vi "SetHFLockIn.vi"(0 "HF Lockin Cluster":T1={"Amplitude"=-inf, "Phase Shift"=-inf, "Frequency"=-inf, "Integration Time"=-inf, "Sensitivity"=-inf} {"Sensitivity" format="%#_g V"; "Integration Time" format="%#_g µs"; "Frequency" format="%#_g kHz"; "Phase Shift" format="%#_g deg"; "Amplitude" format="%#_g V"}, 5 "error in":T2) -> (14 "Output Cluster":T1={"Amplitude"=-inf, "Phase Shift"=-inf, "Frequency"=-inf, "Integration Time"=-inf, "Sensitivity"=-inf} {"Sensitivity" format="%#_g V"; "Integration Time" format="%#_g µs"; "Frequency" format="%#_g kHz"; "Phase Shift" format="%#_g deg"; "Amplitude" format="%#_g V"}, 19 "error out":T2)   [LabVIEW 2016]
doc: "Sets all parameters relevant to the high frequency lock in. The input cluster contains:\n- Amplitude in V (float) [0 to 10]\n- Frequency in kHz (float) [0 to 2000]\n- Sensitivity in V (float) [0 to 20]\n- Phase Shift in deg (float) [0 to 360]\n- Integration Time in us (float) [1 to 1000000]\nBy passing -Inf (float) or -2147483648 (integer) as input values, the corresponding parameter(s) will be read out."
uses:
  Controls/HF-Lockin_Parameters.ctl
  Controls/Error_Out.ctl
  Files_ASC500/DLL/ASC500_RemoteControlV27.dll
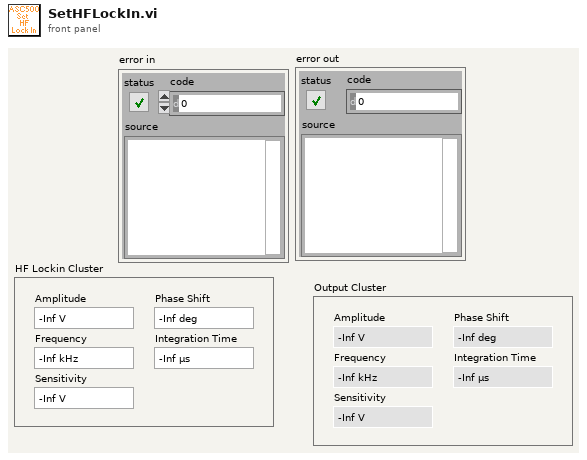
[diagram p1: front panel]
types:
  T1 = typedef "HF-Lockin_Parameters.ctl" = cluster{"Amplitude":sgl, "Phase Shift":sgl, "Frequency":sgl, "Integration Time":sgl, "Sensitivity":sgl}
  T2 = typedef "Error_Out.ctl" = errorcluster
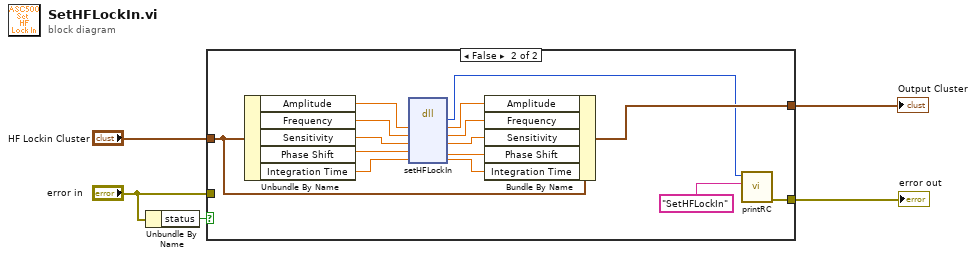
[diagram p0: block diagram]
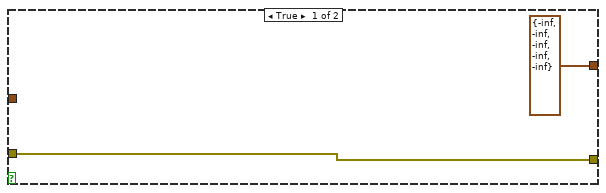
[diagram p2: hidden frame]
diagram:
  n1 = Unbundle By Name("error in") -> ("status"=w5:bool)
  n2 = case shown="False" w5 {
    tunnel: [w6 w10] -> w4
    tunnel: "HF Lockin Cluster" -> [_ w12]
    tunnel: [T1 {"Amplitude"=-inf, "Phase Shift"=-inf, "Frequency"=-inf, "Integration Time"=-inf, "Sensitivity"=-inf} ("HF Lockin Cluster") w11] -> w2
    tunnel: "error in" -> [w6 _]
    frame True {
    }
    frame False {
      n3 = Unbundle By Name(w12) -> ("Amplitude"=w18:sgl, "Frequency"=w19:sgl, "Sensitivity"=w20:sgl, "Phase Shift"=w21:sgl, "Integration Time"=w22:sgl)
      n4 = dll-call lib="G:/SCMOperations/Share/ELE/Produkt Information/ASC500/04 Remote Control/02 development versions/2018Nov06/Files_ASC500/DLL/ASC500_RemoteControlV27.dll" fn="setHFLockIn"("Amplitude"=w18, "Frequency"=w19, "Sensitivity"=w20, "Phase Shift"=w21, "Integration Time"=w22) -> ("return type"=w9:i32, "Amplitude"=w17:sgl, "Frequency"=w16:sgl, "Sensitivity"=w15:sgl, "Phase Shift"=w14:sgl, "Integration Time"=w13:sgl)  [unwired: 3 in, 2 out]
      n5 = Bundle By Name(cluster=w12, "Amplitude"=w17, "Frequency"=w16, "Sensitivity"=w15, "Phase Shift"=w14, "Integration Time"=w13) -> (w11:T1)
      n6 = call "printRC.vi"("additional information"="SetHFLockIn", "RC"=w9) -> ("error out"=w10:T2)  [unwired: 9 in]
    }
  }
  "error out" <- w4
  "Output Cluster" <- w2
